vi "CRYRun Selected Project.vi"(11 "sequence name":string) -> (3 "run state":bool)   [LabVIEW 2013]
uses:
  CRYProject Run Control Global.vi
  Calibration/SubVI/CRYCal Global.vi
  Program/CRYRef nums global.vi
  CRYWindow/SubVI/CRYMain Sub Window Global.vi
  <vilib>/Utility/miscctls.llb/LVRectTypeDef.ctl
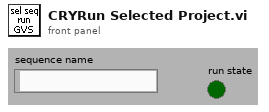
[diagram p1: front panel]
types:
  T1 = typedef "LVRectTypeDef.ctl" = cluster{"Left":i16, "Top":i16, "Right":i16, "Bottom":i16}
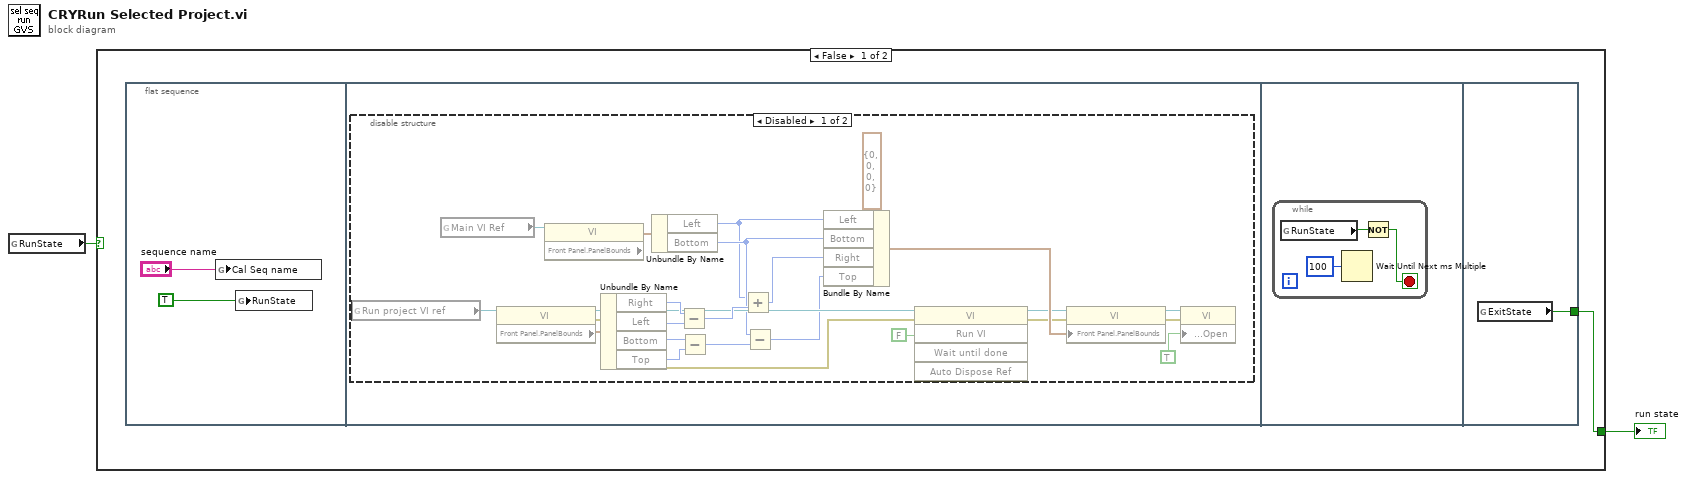
[diagram p0: block diagram]
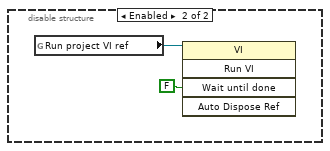
[diagram p2: hidden frame]
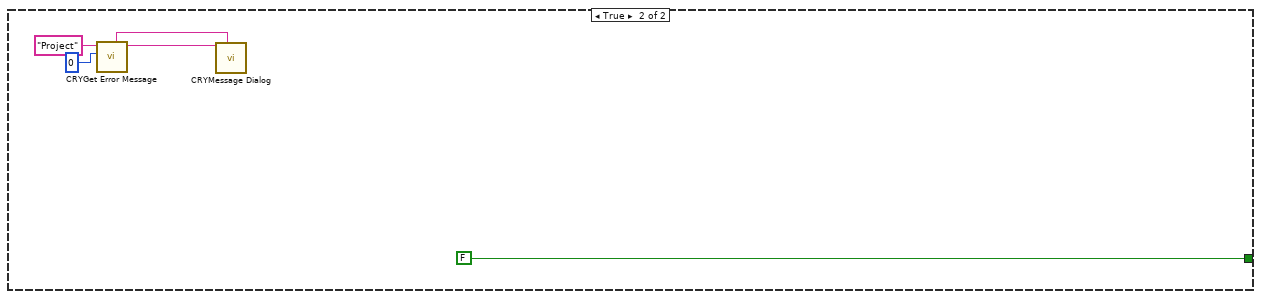
[diagram p3: hidden frame]
diagram:
  n1 = global read "CRYProject Run Control Global.vi" "RunState"() -> (w2:bool)
  n2 = case shown="False" w2 {
    tunnel: [w3 FALSE] -> w1
    frame False {
      n3 = flat-sequence {
        tunnel: [w35] -> w3
        frame #0 {
          n4 = global write "CRYCal Global.vi" "Cal Seq name"("sequence name") -> ()
          n5 = global write "CRYProject Run Control Global.vi" "RunState"(TRUE ("RunState")) -> ()
        }
        frame #1 {
          n6 = disable-structure shown="Disabled" {
            frame Disabled {
              n7 = global read "CRYRef nums global.vi" "Run project VI ref"() -> (w15:refnum<vi>)
              n8 = global read "CRYMain Sub Window Global.vi" "Main VI Ref"() -> (w8:refnum<vi>)
              n9 = property class="VI"(reference=w15) -> (reference out=w16:refnum<vi>, error out=w22:errorcluster, "Front Panel.PanelBounds"=w23:T1)  [unwired: 1 in]
              n10 = property class="VI"(reference=w8) -> ("Front Panel.PanelBounds"=w9:T1)  [unwired: 1 in, 2 out]
              n11 = Unbundle By Name(w23) -> ("Right"=w24:i16, "Left"=w25:i16, "Bottom"=w26:i16, "Top"=w27:i16)
              n12 = Unbundle By Name(w9) -> ("Left"=w10:i16, "Bottom"=w12:i16)
              n13 = Subtract(x=w24, y=w25) -> (x-y=w28:i16)
              n14 = Subtract(x=w26, y=w27) -> (x-y=w29:i16)
              n15 = Add(x=w10, y=w28) -> (x+y=w11:i16)
              n16 = Subtract(x=w12, y=w29) -> (x-y=w13:i16)
              n17 = Bundle By Name(cluster=T1 {"Left"=0, "Top"=0, "Right"=0, "Bottom"=0} ("Front Panel Window:Panel Bounds"), "Left"=w10, "Bottom"=w12, "Right"=w11, "Top"=w13) -> (w21:T1)
              n18 = invoke class="VI" method="Run VI"(reference=w16, error in=w22, "Wait until done"=FALSE ("Wait Until Done")) -> (reference out=w17:refnum<vi>, error out=w19:errorcluster)  [unwired: 2 in, 3 out]
              n19 = property class="VI"(reference=w17, error in=w19, "Front Panel.PanelBounds"=w21) -> (reference out=w18:refnum<vi>, error out=w20:errorcluster)
              n20 = property class="VI"(reference=w18, error in=w20, "Front Panel.Open"=TRUE ("Front Panel Window:Open")) -> ()  [unwired: 2 out]
            }
            frame Enabled {
              n21 = global read "CRYRef nums global.vi" "Run project VI ref"() -> (w30:refnum<vi>)
              n22 = invoke class="VI" method="Run VI"(reference=w30, "Wait until done"=FALSE ("Wait Until Done")) -> ()  [unwired: 3 in, 5 out]
            }
          }
        }
        frame #2 {
          n23 = while {
            stop <- w33 stop-if-true
            n24 = global read "CRYProject Run Control Global.vi" "RunState"() -> (w34:bool)
            n25 = Wait Until Next ms Multiple(millisecond multiple=u32 100) -> ()  [unwired: 1 out]
            n26 = Not(x=w34) -> (.not. x?=w33:bool)
          }
        }
        frame #3 {
          n27 = global read "CRYProject Run Control Global.vi" "ExitState"() -> (w35:bool)
        }
      }
    }
    frame True {
      n28 = call "CRYGet Error Message.vi"("Error No"=0, "Kind"="Project") -> ("Message"=w36:string, "Window Title"=w37:string)  [unwired: 4 in, 4 out]
      n29 = call "CRYMessage Dialog.vi"("Window Title"=w37, "Message Content"=w36) -> ()  [unwired: 8 in, 2 out]
    }
  }
  "run state" <- w1
